vi "ucs.vi"() -> ()   [LabVIEW 2016]
panel:
  out "System Gauge":dbl(knob) scale=0.0..10.0
  out "System Intensity Chart":dbl[][](graph)
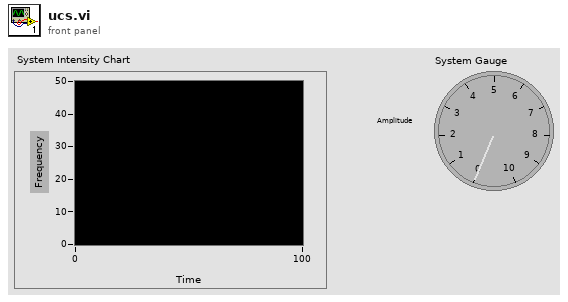
[diagram p1: front panel]
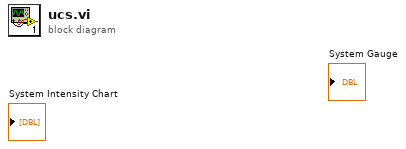
[diagram p0: block diagram]
diagram:
